vi "Do Two Step Build.vi"(8 "error in (no error)":errorcluster, 11 "NI_AB_API_RESTful in":refnum<class "NI_AB_API_RESTful.lvclass">) -> (0 "error out":errorcluster, 2 "GeneratedFiles":path[](array[path]), 3 "NI_AB_API_RESTful out":refnum<class "NI_AB_API_RESTful.lvclass">)   [LabVIEW 2020, in "NI_AB_API_RESTful.lvclass"]
uses:
  <vilib>/AppBuilder/AB_API/RESTful/NI_AB_API_RESTful.lvclass
  <vilib>/AppBuilder/AB_API/RESTful/NI_AB_API_RESTful.lvclass/NI_AB_API_RESTful.ctl
  <vilib>/AppBuilder/AB_API/Targetfile/NI_AB_API_Targetfile.lvclass
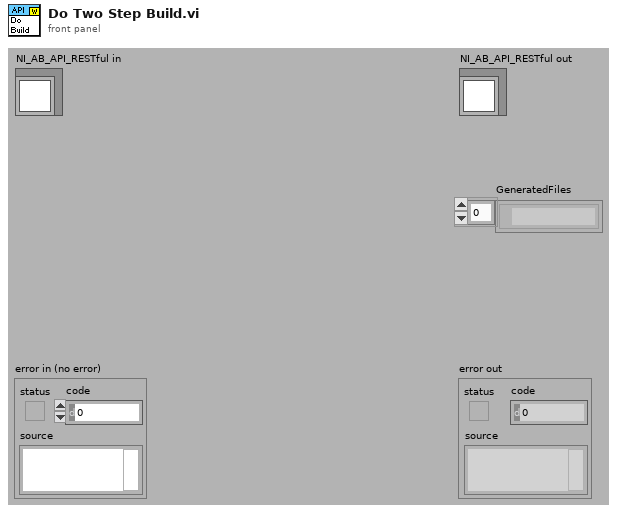
[diagram p1: front panel]
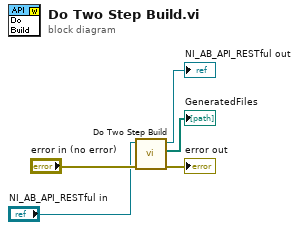
[diagram p0: block diagram]
diagram:
  n1 = call-parent "Do Two Step Build.vi"("error in (no error)"="error in (no error)", "NI_AB_API_Build in"="NI_AB_API_RESTful in") -> ("error out"=→"error out":errorcluster, "GeneratedFiles"=→"GeneratedFiles":path[], "NI_AB_API_Build out"=→"NI_AB_API_RESTful out":refnum<class "NI_AB_API_RESTful.lvclass">)  [unwired: 7 in]
